vi "AtSpectrograph_monitorCommand_standby.vi"(8 "error in (no error)":errorcluster, 11 "command_standby_Ctl":T1) -> (0 "error out":errorcluster, 2 "function return":i32, 3 "command_standby_Ctl out":T1)   [LabVIEW 2016, in "SALLV_AtSpectrograph.lvlib"]
doc: "int AtSpectrograph_shm_monitorCommand_standbyLV(AtSpectrograph_command_standbyLV *command_standby_Ctl );"
uses:
  SALLV_AtSpectrograph.lvlib
  DataTypes/command_standby.ctl
  SALLV_AtSpectrograph.so
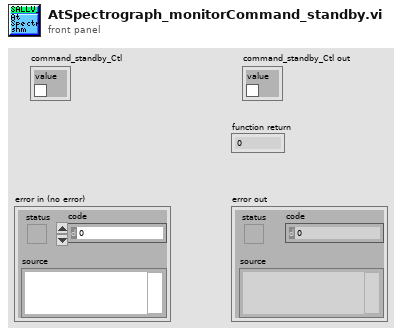
[diagram p1: front panel]
types:
  T1 = typedef "SALLV_AtSpectrograph.lvlib/command_standby.ctl" = cluster{"value":bool}
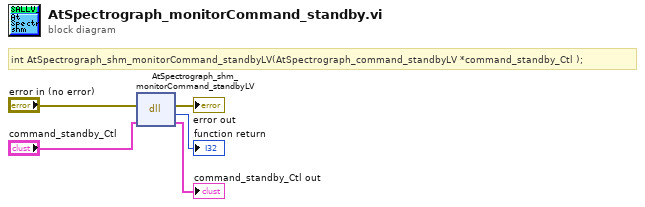
[diagram p0: block diagram]
diagram:
  # "int AtSpectrograph_shm_monitorCommand_standbyLV(AtSpectrograph_command_standbyLV *command_standby_Ctl );"
  n1 = dll-call lib="home/harini/tcs/temp/SALLV_AtSpectrograph/SALLV_AtSpectrograph.*" fn="AtSpectrograph_shm_monitorCommand_standbyLV"(error in="error in (no error)", "command_standby_Ctl"="command_standby_Ctl") -> (error out=→"error out":errorcluster, →"function return":i32, "command_standby_Ctl"=→"command_standby_Ctl out":T1)  [unwired: 2 in, 1 out]
